vi "Preview Test Channel.vi"(8 "error in (no error)":errorcluster, 11 "Test Channel Model in":refnum<class "Test Channel Model.lvclass">) -> (0 "error out":errorcluster, 3 "Test Channel Model out":refnum<class "Test Channel Model.lvclass">)   [LabVIEW 2013, in "Test Channel Model.lvlib" / "Test Channel Model.lvclass"]
uses:
  Test Channel Model.lvclass
  Test Channel Model.lvclass/Test Channel Model.ctl
  Data Accessors/Get Test Node Path.vi
  <vilib>/xml/Load XML File.vi
  <vilib>/xml/Close Reference(Node).vi
  <vilib>/xml/NI_XML.lvlib
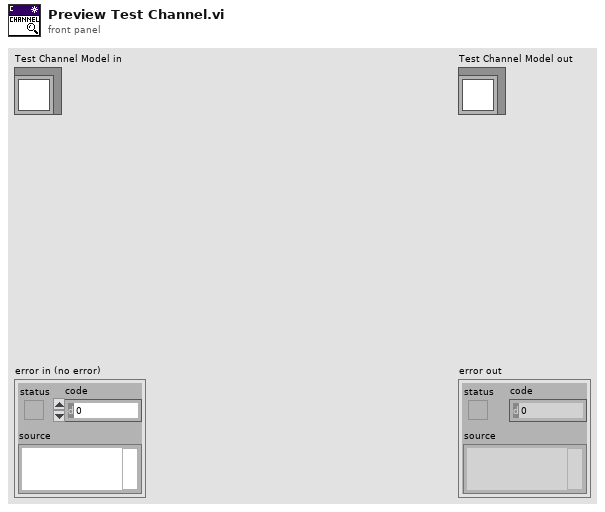
[diagram p1: front panel]
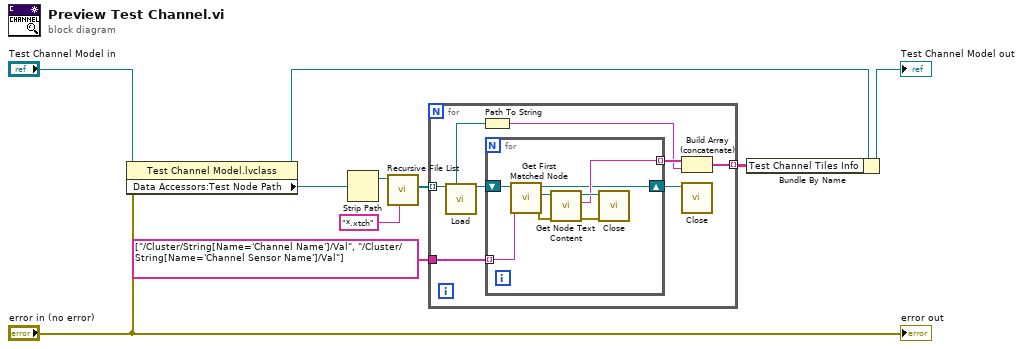
[diagram p0: block diagram]
diagram:
  n1 = property class="Test Channel Model.lvclass"(reference="Test Channel Model in", error in="error in (no error)") -> (reference out=w2:refnum<class "Test Channel Model.lvclass">, "Data Accessors:Test Node Path"=w3:path)  [unwired: 1 out]
  n2 = Strip Path(path=w3) -> (stripped path=w6:path)  [unwired: 1 out]
  n3 = call <vilib>:"Recursive File List.vi"("pattern"="*.xtch", "Folder Path"=w6) -> ("All Files in Dir"=w7:path[])  [unwired: 5 in, 4 out]
  n4 = for {
    tunnel: w7 -> [w14] mode=indexing
    tunnel: string[] ["/Cluster/String[Name='Channel Name']/Val", "/Cluster/String[Name='Channel Sensor Name']/Val"] -> [w16]
    tunnel: [w11] -> w8 mode=indexing
    n5 = call-poly <vilib>:"Load.vi"("path to XML document"=w14) -> ("DOM document out"=w17:refnum<k20>)  [unwired: 12 in, 2 out]
    n6 = Path To String(path=w14) -> (string=w13:string)
    n7 = for {
      shift-right: [w18] -> w12
      shift-left: w17 -> [w25]
      tunnel: w16 -> [w24] mode=indexing
      tunnel: [w21] -> w15 mode=indexing
      n8 = call <vilib>:"Get First Matched Node.vi"("XPath expression"=w24, "node in"=w25) -> ("error out"=w19:errorcluster, "node result"=w23:refnum<k20>, "node out"=w18:refnum<k20>)  [unwired: 7 in]
      n9 = call <vilib>:"Get Node Text Content.vi"("error in (no error)"=w19, "node in"=w23) -> ("error out"=w20:errorcluster, "node text"=w21:string, "node out"=w22:refnum<k20>)  [unwired: 7 in]
      n10 = call-poly <vilib>:"Close.vi"("error in (no error)"=w20, "node"=w22) -> ()  [unwired: 7 in, 1 out]
    }
    n11 = Build Array (concatenate)(w15, w13) -> (w11:string[])
    n12 = call-poly <vilib>:"Close.vi"("node"=w12) -> ()  [unwired: 8 in, 1 out]
  }
  n13 = Bundle By Name(cluster=w2, "Test Channel Tiles Info"=w8) -> (→"Test Channel Model out":refnum<class "Test Channel Model.lvclass">)
  "error out" <- "error in (no error)"
